vi "Set Temperature.vi"(8 "error in (no error)":errorcluster, 11 "Cooler in":refnum<class "Cooler.lvclass">) -> (0 "error out":errorcluster, 3 "Cooler out":refnum<class "Cooler.lvclass">)   [LabVIEW 2018, in "Cooler.lvclass"]
uses:
  Cooler.lvclass
  C:/Users/observer/Desktop/SPARC4_ACS/SPARC4_ACS/Simulated_Cooler/Simulated_Cooler.lvclass
  Simulated_Cooler/Simulated_Cooler.lvclass/Simulated_Cooler.ctl
  Simulated_Cooler/Simulated_Cooler.lvclass
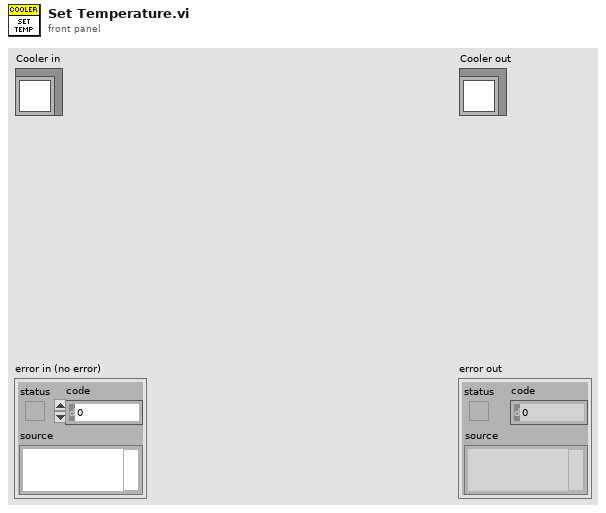
[diagram p1: front panel]
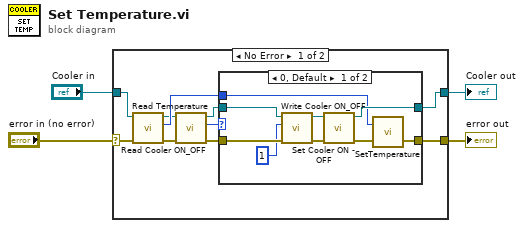
[diagram p0: block diagram]
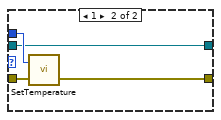
[diagram p2: hidden frame]
diagram:
  n1 = case shown="No Error" "error in (no error)" {
    selector: "error in (no error)" -> [w13 w29]
    tunnel: [w14 w29] -> w2
    tunnel: [w10 w28] -> w3
    tunnel: "Cooler in" -> [w12 w28]
    frame No Error {
      n2 = call-dynamic "Read Temperature.vi"("error in (no error)"=w13, "Cooler in"=w12) -> ("error out"=w8:errorcluster, "Temperature"=w11:i32, "Cooler out"=w9:refnum<class "Cooler.lvclass">)  [unwired: 7 in]
      n3 = call "Read Cooler ON_OFF.vi"("error in (no error)"=w8, "Cooler in"=w9) -> ("error out"=w5:errorcluster, "Cooler ON/OFF"=w7:u8, "Cooler out"=w6:refnum<class "Cooler.lvclass">)  [unwired: 7 in]
      n4 = case shown="0, Default" w7 {
        tunnel: [w17 w27] -> w14
        tunnel: w5 -> [w22 w26]
        tunnel: w11 -> [w15 w25]
        tunnel: w6 -> [w23 w24]
        tunnel: [w18 w24] -> w10
        frame 0, Default {
          n5 = call "Write Cooler ON_OFF.vi"("error in (no error)"=w22, "Cooler ON/OFF"=u8 1, "Cooler in"=w23) -> ("error out"=w19:errorcluster, "Cooler out"=w20:refnum<class "Cooler.lvclass">)  [unwired: 7 in]
          n6 = call-dynamic "Set Cooler ON - OFF.vi"("error in (no error)"=w19, "Cooler in"=w20) -> ("error out"=w16:errorcluster, "Cooler out"=w18:refnum<class "Cooler.lvclass">)  [unwired: 8 in]
          n7 = call <userlib>:"SetTemperature.vi"("error in (no error)"=w16, "temperature"=w15) -> ("error out"=w17:errorcluster)  [unwired: 1 out]
        }
        frame 1 {
          n8 = call <userlib>:"SetTemperature.vi"("error in (no error)"=w26, "temperature"=w25) -> ("error out"=w27:errorcluster)  [unwired: 1 out]
        }
      }
    }
    frame Error {
    }
  }
  "error out" <- w2
  "Cooler out" <- w3
